vi "111_IO.vi"() -> ()   [LabVIEW 2018]
uses:
  Database/Global1.vi
  <vilib>/addons/database/Connection.llb/DB Tools Open Connec (String).vi
  <vilib>/addons/database/Connection.llb/Conn Execute.vi
  <vilib>/addons/database/Recordset.llb/Rec Fetch Recordset Data (R).vi
  <vilib>/addons/database/NI_Database_API.lvlib
panel:
  out "codeid":string
  out "deviceid":string
  out "productid":string
  # "调阀台"
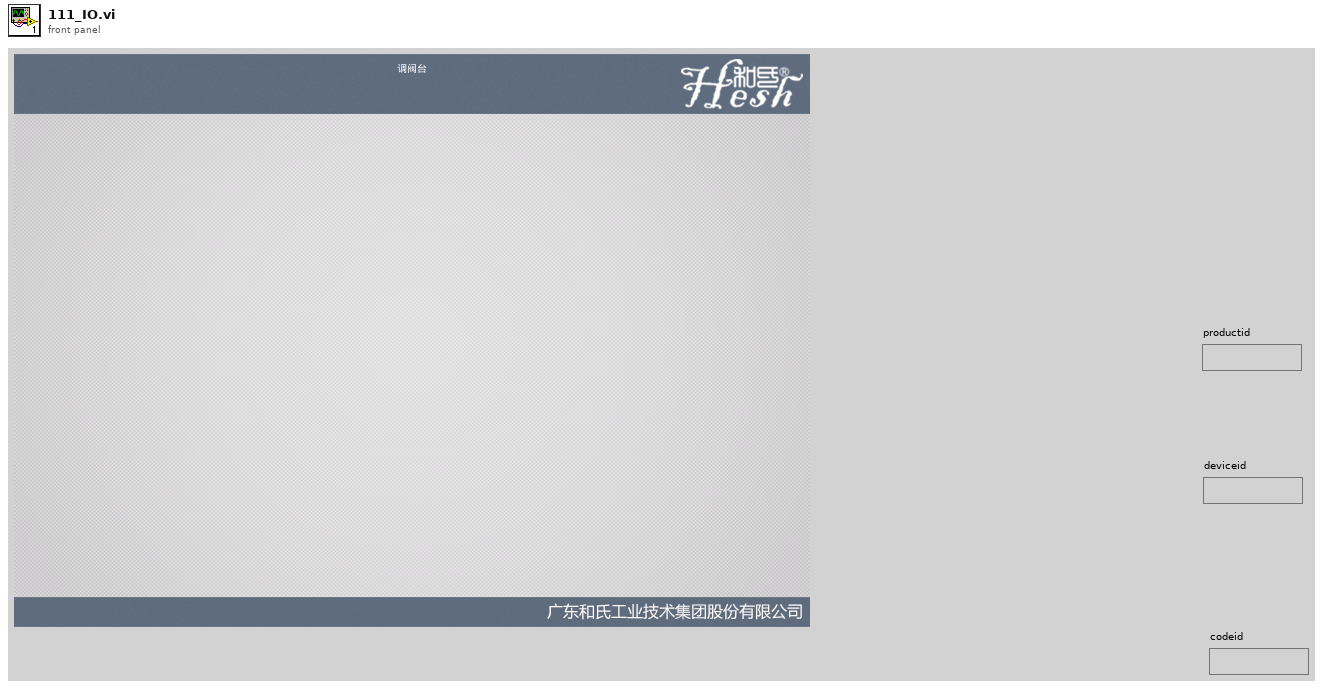
[diagram p1: front panel]
types:
  T1 = typedef "NI_Database_API.lvlib/Conn ObjectReference.ctl" = refnum<k1>
  T2 = typedef "NI_Database_API.lvlib/Rec ObjectReference.ctl" = refnum<k1>
  T3 = cluster{i64, i64, string, sgl, sgl, string, string, string}
  T4 = cluster{i64, i64, string, sgl, sgl, string, string, string}[]
  T5 = cluster{i64, i64, sgl, sgl, string, string, string}
  T6 = cluster{i64, "默认(0 I32)":i64, i64, string, "result string":string}
  T7 = cluster{i64, "默认(0 I32)":i64, i64, string, "result string":string}[]
  T8 = cluster{i64, "默认(0 I32)":i64, string, "result string":string}
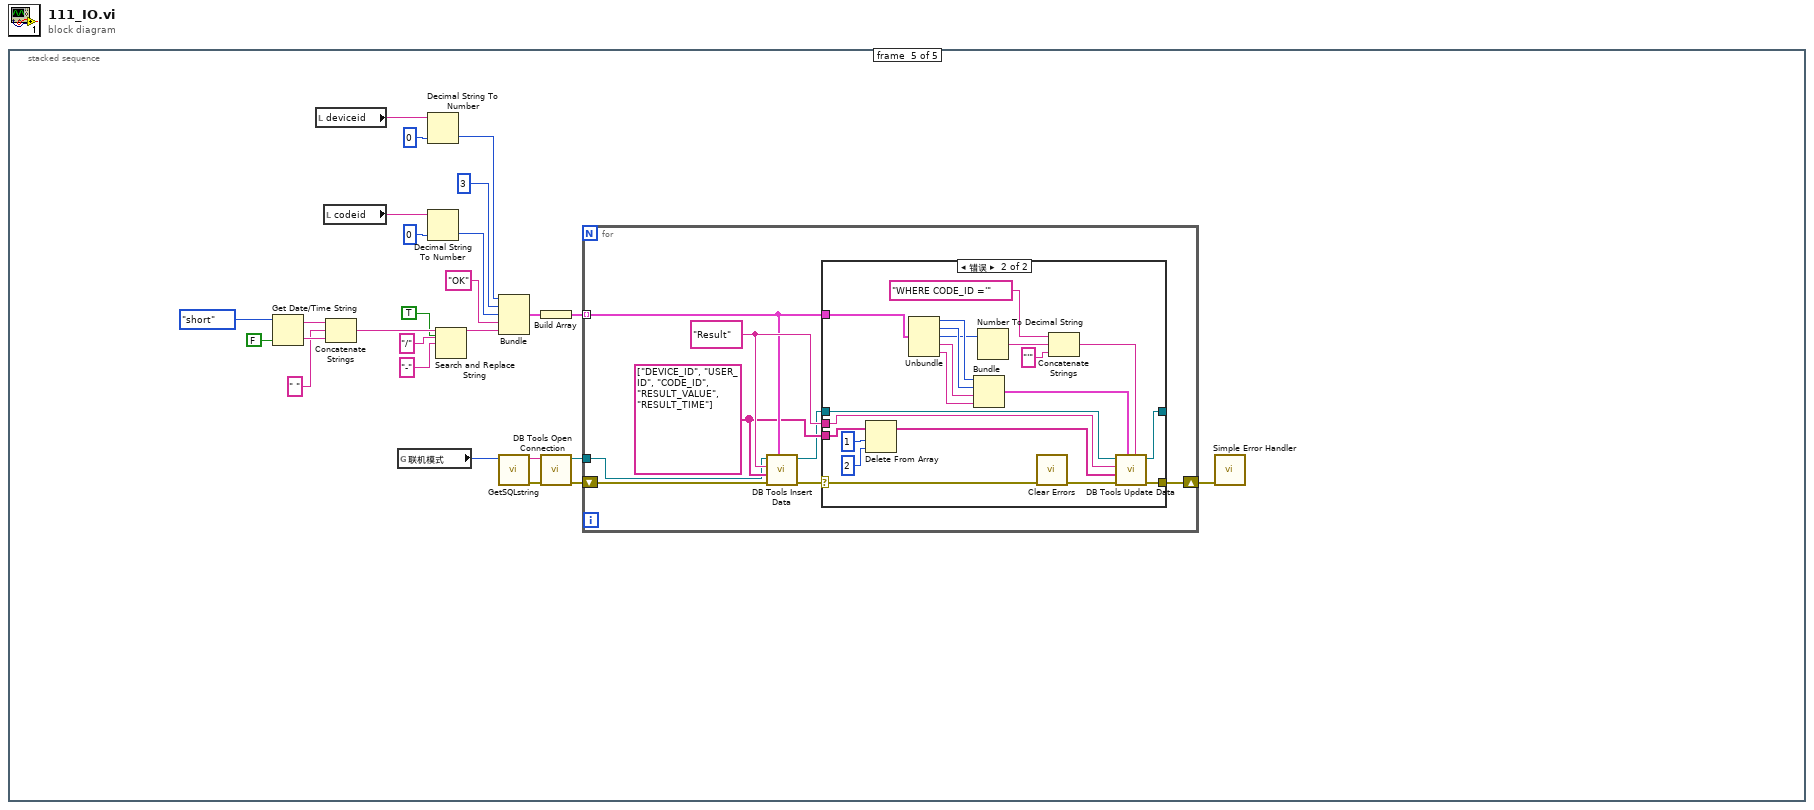
[diagram p0: block diagram]
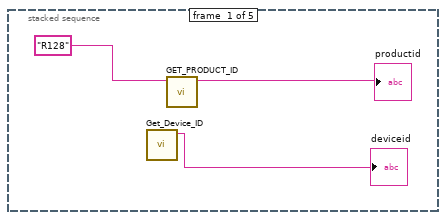
[diagram p2: hidden frame]
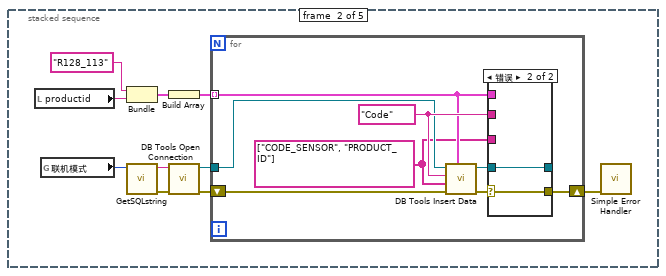
[diagram p3: hidden frame]
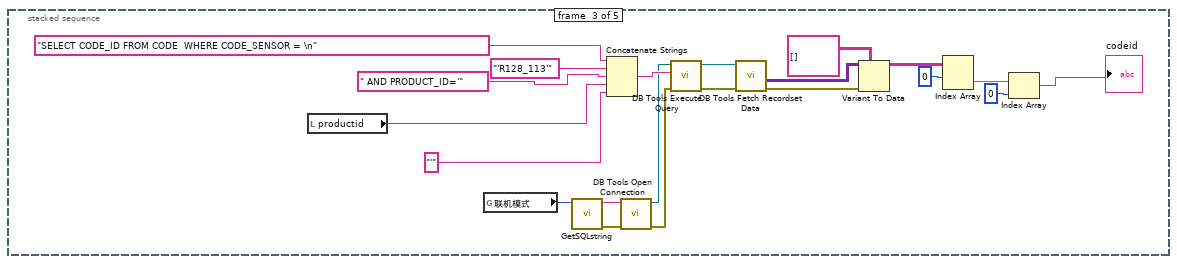
[diagram p5: hidden frame]
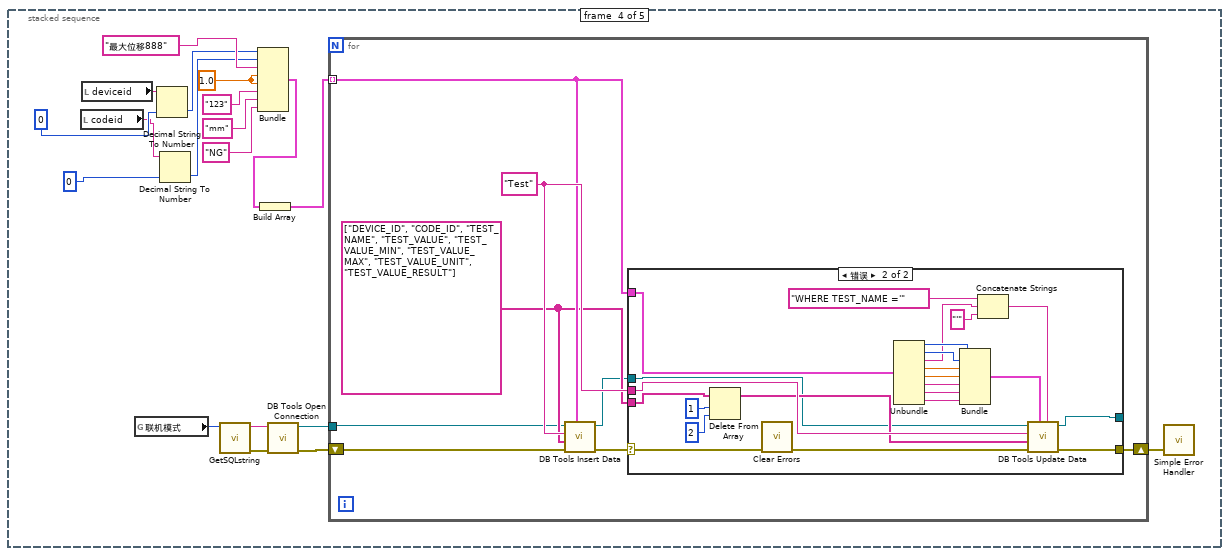
[diagram p6: hidden frame]
diagram:
  n1 = stacked-sequence {
    frame #0 {
      n2 = call "Get_Device_ID.vi"() -> ("Device_ID"=→"deviceid":string)  [unwired: 10 in, 1 out]
      n3 = call "GET_PRODUCT_ID.vi"("PRODFUCT_NAME"="R128") -> ("PRODUCT_ID"=→"productid":string)  [unwired: 10 in]
    }
    frame #1 {
      n4 = local read "productid"() -> (w4:string)
      n5 = global read "Global1.vi" "联机模式"() -> (w12:enum16{"单机", "追溯"})
      n6 = Bundle("R128_113", "productid"=w4) -> (w6:cluster{string, "productid":string})  [unwired: 1 in]
      n7 = call "GetSQLstring.vi"("联机模式"=w12) -> ("错误输出"=w10:errorcluster, "连接字符串"=w11:string)  [unwired: 9 in]
      n8 = Build Array(w6) -> (w5:cluster{string, "productid":string}[])
      n9 = call-poly <vilib>:"DB Tools Open Connection.vi"("error in (no error)"=w10, "connection information"=w11) -> ("error out"=w13:errorcluster, "connection reference"=w9:T1)  [unwired: 6 in]
      n10 = for {
        tunnel: w5 -> [w18] mode=indexing
        tunnel: w9 -> [w17]
        shift-right: [w15] -> w7
        shift-left: w13 -> [w21]
        w14 = string[] ["CODE_SENSOR", "PRODUCT_ID"] ("columns")
        w19 = "Code" ("table")
        n11 = call <vilib>:"DB Tools Insert Data.vi"("data"=w18, "error in (no error)"=w21, "columns"=w14, "table"=w19, "connection reference"=w17) -> ("error out"=w20:errorcluster, "connection reference out"=w16:T1)  [unwired: 5 in]
        n12 = case shown="错误" w20 {
          selector: w20 -> [w22 w24]
          tunnel: w14 -> [_ _]
          tunnel: w16 -> [w23 w25]
          tunnel: w19 -> [_ _]
          tunnel: w18 -> [_ _]
          tunnel: [w23 w25] -> _
          tunnel: [w22 w24] -> w15
          frame No Error {
          }
          frame Error {
          }
        }
      }
      n13 = call <vilib>:"Simple Error Handler.vi"("error in (no error)"=w7) -> ()  [unwired: 4 in, 5 out]
    }
    frame #2 {
      n14 = local read "productid"() -> (w27:string)
      n15 = global read "Global1.vi" "联机模式"() -> (w46:enum16{"单机", "追溯"})
      n16 = call "GetSQLstring.vi"("联机模式"=w46) -> ("错误输出"=w44:errorcluster, "连接字符串"=w45:string)  [unwired: 9 in]
      n17 = Concatenate Strings("SELECT CODE_ID FROM CODE  WHERE CODE_SENSOR = \n" ("table"), "'R128_113'" ("字符串"), " AND PRODUCT_ID='" ("字符串"), w27, "'" ("字符串")) -> (w43:string)
      n18 = call-poly <vilib>:"DB Tools Open Connection.vi"("error in (no error)"=w44, "connection information"=w45) -> ("error out"=w37:errorcluster, "connection reference"=w38:T1)  [unwired: 6 in]
      n19 = call-poly <vilib>:"DB Tools Execute Query.vi"("error in (no error)"=w37, "SQL query"=w43, "connection reference"=w38) -> ("error out"=w41:errorcluster, "recordset reference"=w42:T2)  [unwired: 5 in]
      n20 = call-poly <vilib>:"DB Tools Fetch Recordset Data.vi"("error in (no error)"=w41, "recordset reference"=w42) -> ("error out"=w33:errorcluster, "recordset data"=w40:variant[][])  [unwired: 3 in, 1 out]
      n21 = Variant To Data(error in=w33, type=string[][] [], Variant=w40) -> (data=w32:string[][])  [unwired: 1 out]
      n22 = Index Array(array=w32, index (row)=0 ("索引 (行)")) -> (element=w30:string[])  [unwired: 1 in]
      n23 = Index Array(array=w30, index=0 ("索引 (行)")) -> (element=→"codeid":string)
    }
    frame #3 {
      w56 = sgl 1.0
      n24 = local read "codeid"() -> (w48:string)
      n25 = local read "deviceid"() -> (w52:string)
      n26 = global read "Global1.vi" "联机模式"() -> (w64:enum16{"单机", "追溯"})
      n27 = Decimal String To Number(string=w52, default (0L)=i64 0 ("默认(0 I32)")) -> (number=w50:i64)  [unwired: 1 in, 1 out]
      n28 = Decimal String To Number(string=w48, default (0L)=i64 0 ("默认(0 I32)")) -> (number=w49:i64)  [unwired: 1 in, 1 out]
      n29 = call "GetSQLstring.vi"("联机模式"=w64) -> ("错误输出"=w62:errorcluster, "连接字符串"=w63:string)  [unwired: 9 in]
      n30 = Bundle(w50, w49, "最大位移888", w56, w56, "123", "mm", "NG") -> (w54:T3)  [unwired: 1 in]
      n31 = Build Array(w54) -> (w53:T4)
      n32 = call-poly <vilib>:"DB Tools Open Connection.vi"("error in (no error)"=w62, "connection information"=w63) -> ("error out"=w65:errorcluster, "connection reference"=w59:T1)  [unwired: 6 in]
      n33 = for {
        tunnel: w53 -> [w70] mode=indexing
        tunnel: w59 -> [w68]
        shift-right: [w66] -> w55
        shift-left: w65 -> [w73]
        w69 = string[] ["DEVICE_ID", "CODE_ID", "TEST_NAME", "TEST_VALUE", "TEST_VALUE_MIN", "TEST_VALUE_MAX", "TEST_VALUE_UNIT", "TEST_VALUE_RESULT"] ("columns")
        w71 = "Test" ("table")
        n34 = call <vilib>:"DB Tools Insert Data.vi"("data"=w70, "error in (no error)"=w73, "columns"=w69, "table"=w71, "connection reference"=w68) -> ("error out"=w72:errorcluster, "connection reference out"=w67:T1)  [unwired: 5 in]
        n35 = case shown="错误" w72 {
          selector: w72 -> [w74 w97]
          tunnel: w69 -> [_ w94]
          tunnel: w67 -> [w75 w78]
          tunnel: w71 -> [_ w98]
          tunnel: w70 -> [_ w88]
          tunnel: [w75 w77] -> _
          tunnel: [w74 w76] -> w66
          frame No Error {
          }
          frame Error {
            n36 = Delete From Array(array=w94, length=1 ("长度"), index=2 ("索引")) -> (array with subset deleted=w95:string[])  [unwired: 1 out]
            n37 = call <vilib>:"Clear Errors.vi"("error in (no error)"=w97) -> ("error out"=w96:errorcluster)  [unwired: 5 in, 1 out]
            n38 = Unbundle(w88) -> (w87:i64, w86:i64, w79:string, w85:sgl, w84:sgl, w83:string, w82:string, w81:string)
            n39 = Bundle(w87, w86, w85, w84, w83, w82, w81) -> (w80:T5)  [unwired: 1 in]
            n40 = Concatenate Strings("WHERE TEST_NAME ='" ("condition"), w79, "'") -> (w90:string)
            n41 = call <vilib>:"DB Tools Update Data.vi"("condition"=w90, "data"=w80, "error in (no error)"=w96, "columns"=w95, "table"=w98, "connection reference"=w78) -> ("error out"=w76:errorcluster, "connection reference out"=w77:T1)  [unwired: 4 in]
          }
        }
      }
      n42 = call <vilib>:"Simple Error Handler.vi"("error in (no error)"=w55) -> ()  [unwired: 4 in, 5 out]
    }
    frame #4 {
      n43 = Get Date/Time String(date format (0)=enum16{"short", "long", "abbreviated"}."short" ("日期格式(0)"), want seconds? (F)=FALSE ("需要秒？(F)")) -> (date string=w106:string, time string=w105:string)  [unwired: 1 in]
      n44 = local read "deviceid"() -> (w115:string)
      n45 = local read "codeid"() -> (w112:string)
      n46 = Concatenate Strings(w106, " " ("字符串"), w105) -> (w102:string)
      n47 = global read "Global1.vi" "联机模式"() -> (w123:enum16{"单机", "追溯"})
      n48 = Decimal String To Number(string=w115, default (0L)=i64 0 ("默认(0 I32)")) -> (number=w113:i64)  [unwired: 1 in, 1 out]
      n49 = Decimal String To Number(string=w112, default (0L)=i64 0 ("默认(0 I32)")) -> (number=w110:i64)  [unwired: 1 in, 1 out]
      n50 = Search and Replace String(replace all?=TRUE ("替换全部？(F)"), input string=w102, search string="/" ("替换字符串(\"\")"), replace string="-" ("替换字符串(\"\")")) -> (result string=w103:string)  [unwired: 4 in, 3 out]
      n51 = Bundle(w113, "默认(0 I32)"=i64 3, w110, "OK", "result string"=w103) -> (w117:T6)  [unwired: 1 in]
      n52 = call "GetSQLstring.vi"("联机模式"=w123) -> ("错误输出"=w121:errorcluster, "连接字符串"=w122:string)  [unwired: 9 in]
      n53 = Build Array(w117) -> (w116:T7)
      n54 = call-poly <vilib>:"DB Tools Open Connection.vi"("error in (no error)"=w121, "connection information"=w122) -> ("error out"=w124:errorcluster, "connection reference"=w120:T1)  [unwired: 6 in]
      n55 = for {
        tunnel: w116 -> [w129] mode=indexing
        tunnel: w120 -> [w127]
        shift-right: [w125] -> w118
        shift-left: w124 -> [w132]
        w128 = string[] ["DEVICE_ID", "USER_ID", "CODE_ID", "RESULT_VALUE", "RESULT_TIME"] ("columns")
        w130 = "Result" ("table")
        n56 = call <vilib>:"DB Tools Insert Data.vi"("data"=w129, "error in (no error)"=w132, "columns"=w128, "table"=w130, "connection reference"=w127) -> ("error out"=w131:errorcluster, "connection reference out"=w126:T1)  [unwired: 5 in]
        n57 = case shown="错误" w131 {
          selector: w131 -> [w133 w154]
          tunnel: w128 -> [_ w151]
          tunnel: w126 -> [w134 w139]
          tunnel: w130 -> [_ w155]
          tunnel: w129 -> [_ w145]
          tunnel: [w134 w138] -> _
          tunnel: [w133 w137] -> w125
          frame No Error {
          }
          frame Error {
            n58 = Delete From Array(array=w151, length=1 ("长度"), index=2 ("索引")) -> (array with subset deleted=w152:string[])  [unwired: 1 out]
            n59 = Unbundle(w145) -> (w144:i64, "默认(0 I32)"=w143:i64, w135:i64, w142:string, "result string"=w141:string)
            n60 = Bundle(w144, "默认(0 I32)"=w143, w142, "result string"=w141) -> (w140:T8)  [unwired: 1 in]
            n61 = Number To Decimal String(number=w135) -> (decimal integer string=w136:string)  [unwired: 1 in]
            n62 = call <vilib>:"Clear Errors.vi"("error in (no error)"=w154) -> ("error out"=w153:errorcluster)  [unwired: 5 in, 1 out]
            n63 = Concatenate Strings("WHERE CODE_ID ='" ("condition"), w136, "'") -> (w147:string)
            n64 = call <vilib>:"DB Tools Update Data.vi"("condition"=w147, "data"=w140, "error in (no error)"=w153, "columns"=w152, "table"=w155, "connection reference"=w139) -> ("error out"=w137:errorcluster, "connection reference out"=w138:T1)  [unwired: 4 in]
          }
        }
      }
      n65 = call <vilib>:"Simple Error Handler.vi"("error in (no error)"=w118) -> ()  [unwired: 4 in, 5 out]
    }
  }
